vi "Init.vi"(6 "Carrier(13560)Hz":dbl=13560.0, 8 "error in (no error)":errorcluster, 10 "Sett data":T1={"Filter"=4, "Gain"=4.0, "Bit rate"=4.0, "ISO/IEC w "=enum."14443 Type A", "BI"={"R"=0.0, "C"=0.0, "L"=0.0}, "BM"={"R"=0.0, "C"=0.0, "L"=0.0}, "M"={"Метка"=4, "Считыветель"=4}, "Type noise"=enum."Гауссовский шум", "Link"=enum."UPLINK", "Noise attenuator"=0.0, "Signal gain"=1.0, "Distance"=0.0} {"Distance" scale=0.0..10.0; "Signal gain" min=1.0 max=100.0 step=1.0 scale=1.0..30.0; "Noise attenuator" scale=0.01..1.01; "M"."Считыветель" min=4 max=128 step=4; "M"."Метка" min=4 max=128 step=4; "Bit rate" min=4.0 max=128.0 step=4.0; "Gain" min=4.0 max=128.0 step=4.0; "Filter" min=4 max=128 step=4}, 11 "RFID system in":refnum<class "RFID system.lvclass">) -> (0 "error out":errorcluster, 3 "RFID system out":refnum<class "RFID system.lvclass">)   [LabVIEW 2019, in "RFID system.lvclass"]
uses:
  RFID system.lvclass
  TypeDef/Sett data.ctl
  TypeDef/ISO.ctl
  TypeDef/Noise.ctl
  TypeDef/Link.ctl
  RFID system.lvclass/RFID system.ctl
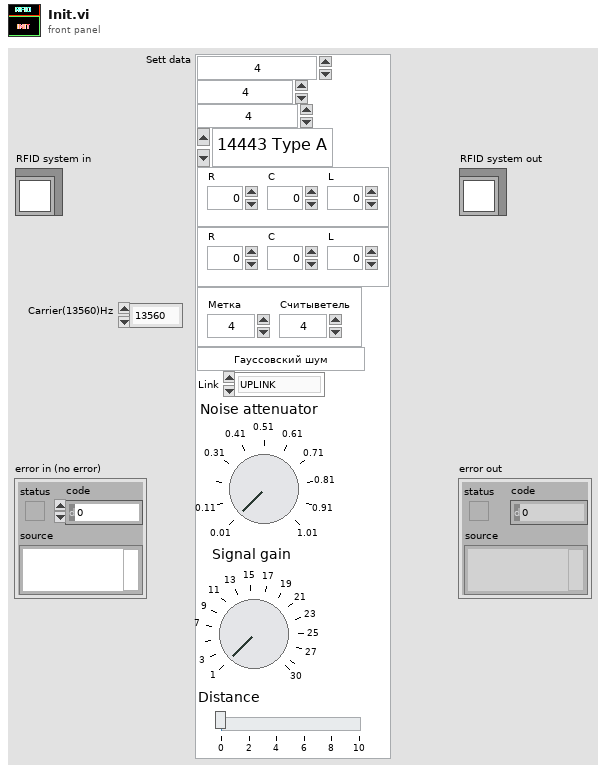
[diagram p1: front panel]
types:
  T1 = typedef "Sett data.ctl" = cluster{"Filter":i32, "Gain":dbl, "Bit rate":dbl, "ISO/IEC w ":T2, "BI":cluster{"R":dbl, "C":dbl, "L":dbl}, "BM":cluster{"R":dbl, "C":dbl, "L":dbl}, "M":cluster{"Метка":i64, "Считыветель":i64}, "Type noise":T3, "Link":T4, "Noise attenuator":dbl, "Signal gain":dbl, "Distance":dbl}
  T2 = typedef "ISO.ctl" = enum16{"14443 Type A", "14443 Type B", "Felica", "15693"}
  T3 = typedef "Noise.ctl" = enum16{"Гауссовский шум", "Белый шум"}
  T4 = typedef "Link.ctl" = enum16{"UPLINK", "DOWNLINK"}
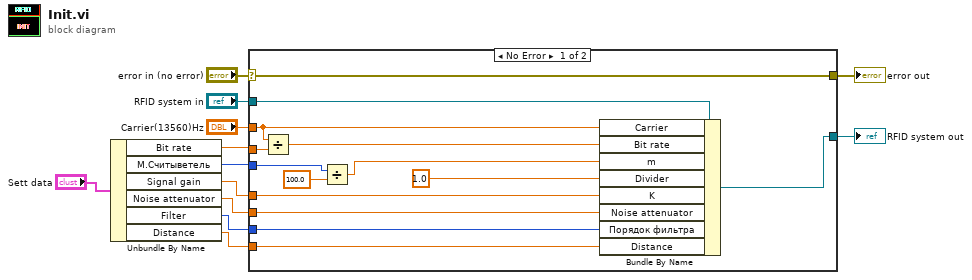
[diagram p0: block diagram]
diagram:
  n1 = Unbundle By Name("Sett data") -> ("Bit rate"=w2:dbl, "M.Считыветель"=w3:i64, "Signal gain"=w4:dbl, "Noise attenuator"=w5:dbl, "Filter"=w6:i32, "Distance"=w1:dbl)
  n2 = case shown="No Error" "error in (no error)" {
    selector: "error in (no error)" -> [w21 w28]
    tunnel: [w21 w28] -> w11
    tunnel: [w25 w27] -> w9
    tunnel: "RFID system in" -> [w26 w27]
    tunnel: "Carrier(13560)Hz" -> [w24 _]
    tunnel: w2 -> [w23 _]
    tunnel: w3 -> [w18 _]
    tunnel: w4 -> [w16 _]
    tunnel: w5 -> [w15 _]
    tunnel: w6 -> [w14 _]
    tunnel: w1 -> [w13 _]
    frame No Error {
      n3 = Divide(x=w24, y=w23) -> (x/y=w22:dbl)
      n4 = Divide(x=w18, y=100.0) -> (x/y=w19:dbl)
      n5 = Bundle By Name(cluster=w26, "Carrier"=w24, "Bit rate"=w22, "m"=w19, "Divider"=1.0, "K"=w16, "Noise attenuator"=w15, "Порядок фильтра"=w14, "Distance"=w13) -> (w25:refnum<class "RFID system.lvclass">)
    }
    frame Error {
    }
  }
  "error out" <- w11
  "RFID system out" <- w9
